vi "parseDataBooleanArray.vi"(8 "error in (no error)":errorcluster, 10 "Length":i32, 11 "U8ArrayParserAutoIndexing in":refnum<class "U8ArrayParserAutoIndexing.lvclass">) -> (0 "error out":errorcluster, 2 "Data":bool[](array[boolean]), 3 "U8ArrayParserAutoIndexing out":refnum<class "U8ArrayParserAutoIndexing.lvclass">)   [LabVIEW 2016, in "RTUtilities.lvlib" / "U8ArrayParserAutoIndexing.lvclass"]
uses:
  U8ArrayParserAutoIndexing.lvclass
  U8ArrayParserAutoIndexing.lvclass/U8ArrayParserAutoIndexing.ctl
  U8ArrayParser/U8ArrayParserManualIndexing.lvclass
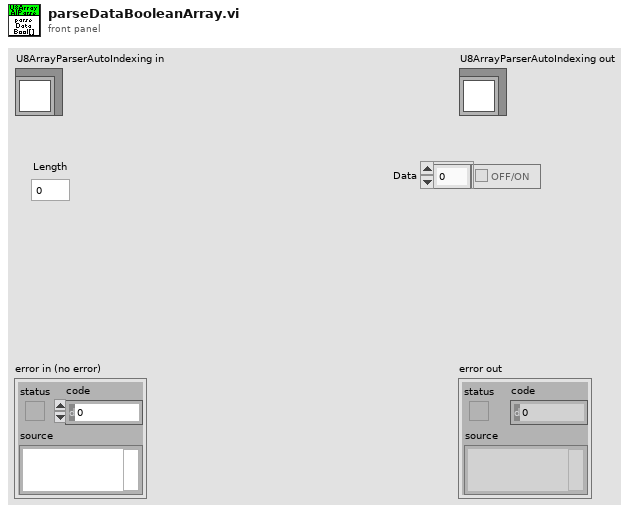
[diagram p1: front panel]
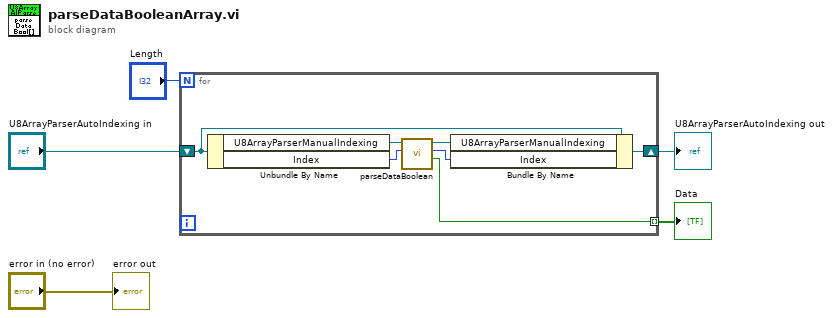
[diagram p0: block diagram]
diagram:
  n1 = for {
    N: "Length" -> [_]
    shift-right: [w11] -> w3
    shift-left: "U8ArrayParserAutoIndexing in" -> [w12]
    tunnel: [w6] -> w2 mode=indexing
    n2 = Unbundle By Name(w12) -> ("U8ArrayParserManualIndexing"=w10:refnum<class "U8ArrayParserManualIndexing.lvclass">, "Index"=w9:i32)
    n3 = call "parseDataBoolean.vi"("Index"=w9, "U8ArrayParserManualIndexing in"=w10) -> ("Data"=w6:bool, "Index out"=w7:i32, "U8ArrayParserManualIndexing out"=w8:refnum<class "U8ArrayParserManualIndexing.lvclass">)  [unwired: 6 in, 1 out]
    n4 = Bundle By Name(cluster=w12, "U8ArrayParserManualIndexing"=w8, "Index"=w7) -> (w11:refnum<class "U8ArrayParserAutoIndexing.lvclass">)
  }
  "U8ArrayParserAutoIndexing out" <- w3
  "Data" <- w2
  "error out" <- "error in (no error)"
